vi "Delete CD Node.vi"(8 "error in":errorcluster, 11 "Tag":string) -> (0 "error out":errorcluster, 1 "Is Enum Property":bool, 4 "Deleted?":bool)   [LabVIEW 2025]
uses:
  <resource>/objmgr/DOMUserDefRef.rc
  Types/TD NodeRef Map Action.ctl
  Types/CD NodeRef Map Action.ctl
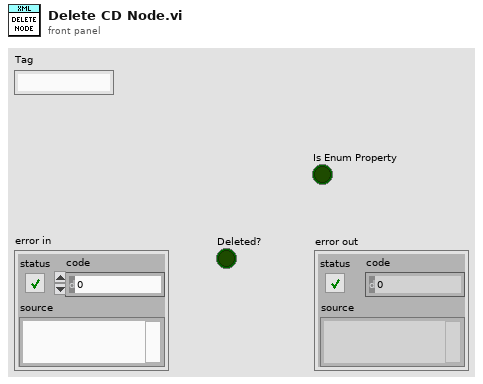
[diagram p1: front panel]
types:
  T1 = typedef "CD NodeRef Map Action.ctl" = enum16{"Init", "Add XMLNodeRef", "Update ParentName", "Delete XMLNodeRef", "Get All Keys", "Get", "skip"}
  T2 = typedef "TD NodeRef Map Action.ctl" = enum16{"Init", "Add XMLNodeRef", "Delete XMLNodeRef", "Add TDNodeRefs", "Delete TDNodeRefs", "Clear TDNodeRefs", "Add ChildXMLNodeRef", "Delete ChildXMLNodeRef", "Get All Keys", "Update ParentName", "Get", "skip"}
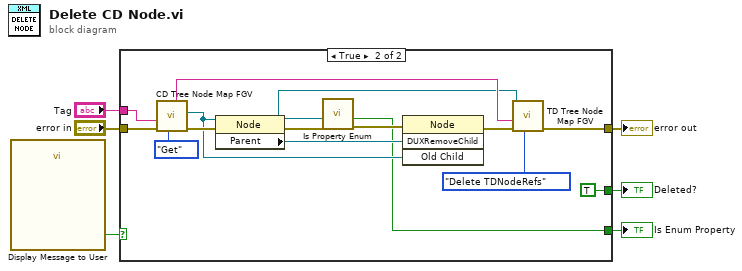
[diagram p0: block diagram]
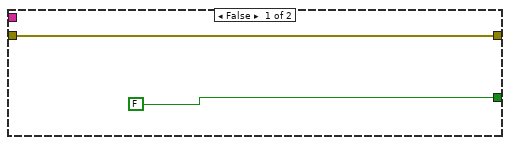
[diagram p2: hidden frame]
diagram:
  n1 = call "Display Message to User"() -> ("Yes"=w4:bool)  [unwired: 10 in, 1 out]
  n2 = case shown="True" w4 {
    tunnel: [w7 w23] -> w3
    tunnel: [FALSE TRUE] -> w6
    tunnel: "Tag" -> [_ w21]
    tunnel: "error in" -> [w7 w16]
    tunnel: [_ w9] -> w1
    frame False {
    }
    frame True {
      n3 = call "CD Tree Node Map FGV.vi"("Action"=CD_NodeRef_Map_Action."Get", "error in"=w16, "Node Name"=w21) -> ("error out"=w19:errorcluster, "Node Reference"=w15:refnum<k20>, "Parent Name out"=w13:string)  [unwired: 4 in, 2 out]
      n4 = property class="Node"(reference=w15, error in=w19) -> (reference out=w10:refnum<k20>, error out=w12:errorcluster, "Parent"=w18:refnum<k20>)
      n5 = call "Is Property Enum.vi"("error in"=w12, "Node"=w10) -> ("error out"=w11:errorcluster, "Is Enum Property"=w9:bool)  [unwired: 7 in, 1 out]
      n6 = invoke class="Node" method="DUXRemoveChild"(reference=w18, error in=w11, "Old Child"=w15) -> (error out=w14:errorcluster)  [unwired: 1 in, 3 out]
      n7 = call "TD Tree Node Map FGV.vi"("Action"=TD_NodeRef_Map_Action."Delete TDNodeRefs", "error in"=w14, "Node Name"=w13, "Attribute Node"=w10) -> ("error out"=w23:errorcluster)  [unwired: 2 in, 5 out]
    }
  }
  "Deleted?" <- w6
  "error out" <- w3
  "Is Enum Property" <- w1
